vi "SM_S700_Serial_String_#AL.vi"(8 "error in (no error)":errorcluster, 11 "read buffer":string) -> (0 "error out":errorcluster, 2 "pump":bool, 3 "timestamp":timestamp)   [LabVIEW 2011]
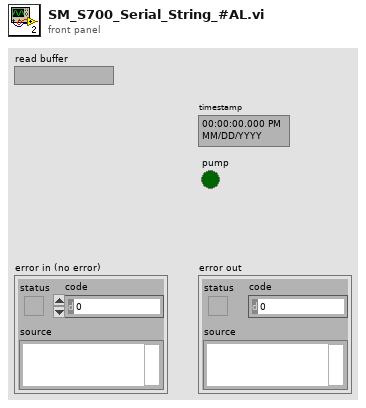
[diagram p1: front panel]
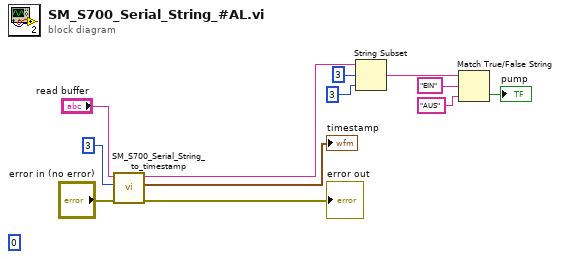
[diagram p0: block diagram]
diagram:
  (unwired) u32 0 ("initial scan location 2")
  n1 = call "SM_S700_Serial_String_to_timestamp.vi"("error in (no error)"="error in (no error)", "initial scan location"=u32 3, "read buffer"="read buffer") -> ("error out"=→"error out":errorcluster, "Time Stamp"=→"timestamp":timestamp, "String"=w6:string)  [unwired: 6 in]
  n2 = String Subset(string=w6, offset (0)=3, length (rest)=3 ("length (rest)")) -> (substring=w5:string)
  n3 = Match True/False String(2:"AUS" ("false string"), 3:"EIN" ("true string"), 4:w5) -> (0:→"pump":bool)  [unwired: 1 out]
